vi "Dispose Report.vi"(0 "report in":refnum<class "NI_report.lvclass">, 5 "wait until printing completed? (T)":bool=TRUE, 9 "save changes? (F)":bool, 11 "error in (no error)":errorcluster, 12 "close report? (T)":bool=TRUE) -> (15 "error out":errorcluster)   [LabVIEW 2020, in "NI_report.lvclass"]
doc: "Closes the report and releases its interface, which saves memory."
uses:
  <vilib>/Utility/NIReport.llb/NI_report.lvclass
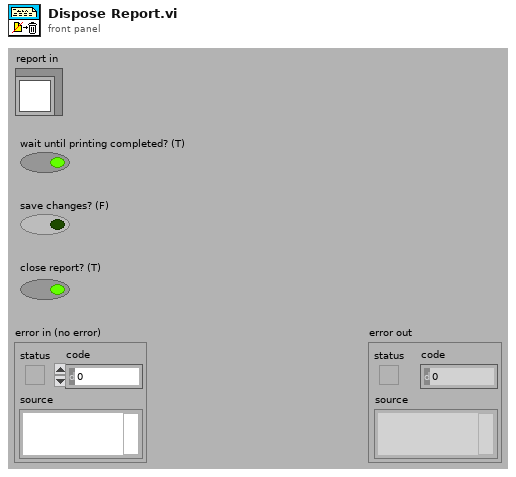
[diagram p1: front panel]
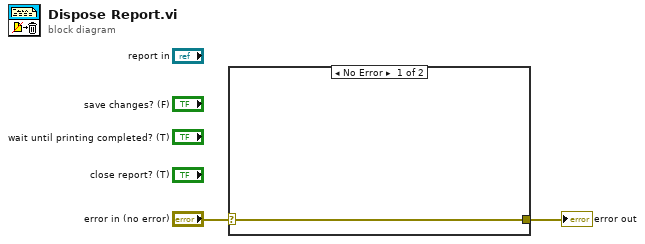
[diagram p0: block diagram]
diagram:
  n1 = case shown="No Error" "error in (no error)" {
    selector: "error in (no error)" -> [w3 w4]
    tunnel: [w3 w4] -> w1
    frame No Error {
    }
    frame Error {
    }
  }
  "error out" <- w1
